vi "SVPO TDMS Write SGL Array (1 Ch).vi"(0 "tdms file":refnum<k34>, 1 "write channel properties? (T)":bool=TRUE, 5 "group name in":string="Waveform", 7 "channel name in":string="Channel0", 9 "scaled signal [EU]":sgl[](array[numeric]), 11 "sampling rate [Hz]":dbl=1.0, 12 "unit label":string) -> (4 "tdms file out":refnum<k34>, 6 "group name out":string, 8 "channel name out":string)   [LabVIEW 2017]
doc: "Writes single-precision waveform or scaled array data to the specified .tdms file in a format specific to the polymorphic instance. Use this VI on embedded targets that have limited computational resources. Wire data to the <B>scaled signal [EU]</B> input to determine the polymorphic instance to use or manually select the instance."
uses:
  <vilib>/addons/_NISVFA/_Shared subVIs/Controls/NI Channel Properties.ctl
  <vilib>/addons/_NISVFA/_Shared subVIs/Controls/LV Datatypes.ctl
  <vilib>/addons/_NISVFA/_Shared subVIs/Controls/svc_X-Axis Units.ctl
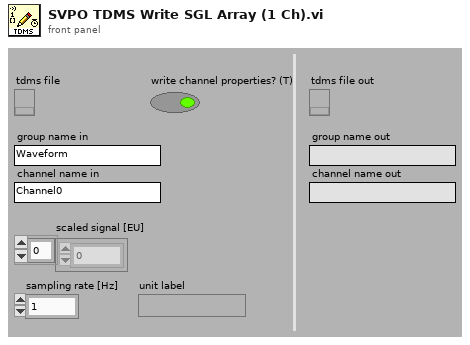
[diagram p1: front panel]
types:
  T1 = typedef "NI Channel Properties.ctl" = u16
  T2 = typedef "svc_X-Axis Units.ctl" = u16
  T3 = typedef "LV Datatypes.ctl" = i32
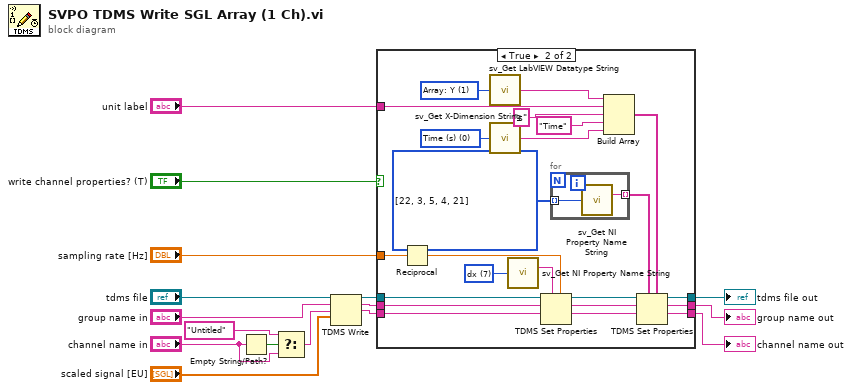
[diagram p0: block diagram]
diagram:
  n1 = Empty String/Path?(string/path="channel name in") -> (empty?=w16:bool)
  n2 = Select(t="Untitled" ("channel name"), s=w16, f="channel name in") -> (s? t:f=w8:string)
  n3 = TDMS Write(0:"tdms file", 5:"group name in", 7:w8, 9:"scaled signal [EU]") -> (4:w13:refnum<k34>, 6:w11:string, 8:w7:string)  [unwired: 2 in, 1 out]
  n4 = case shown="True" "write channel properties? (T)" {
    tunnel: [w19 w42] -> w5
    tunnel: w7 -> [w17 w39]
    tunnel: w11 -> [w18 w40]
    tunnel: w13 -> [w19 w41]
    tunnel: [w18 w33] -> w4
    tunnel: [w17 w34] -> w3
    tunnel: "sampling rate [Hz]" -> [_ w36]
    tunnel: "unit label" -> [_ w22]
    frame False {
    }
    frame True {
      w23 = T1[] [22, 3, 5, 4, 21] items=["Channel name", "Channel description", "Y-axis label", "Y-axis unit string", "X-axis label", "X-axis unit string", "x0", "dx", "Number of samples", "X channel", "Filter settled", "dB reference", "Window", "Window parameter", "Window size", "FFT size", "Peak units", "Spectrum type", "Magnitude scale", "Spectral density", "Sensor sensitivity (mV/EU)", "X-axis domain", "LabVIEW datatype"]
      w28 = T2 0 items=["Time (s)"=0, "Frequency-CB (Hz)"=1, "Frequency-CPB (Hz)"=1248, "Frequency-Arbitrary (Hz)"=2357, "Quefrency (s)"=2, "Revolutions (rev)"=3, "Order"=4, "Speed (RPM)"=11, "Speed (rad/s)"=21, "Index"=65535] ("x-axis units")
      w29 = T3 1 items=["String"=-2, "Boolean"=-1, "Scalar: y"=0, "Array: Y"=1, "Waveform: t0, dt, Y, variant"=2, "Cluster: x0, dx, Y"=3, "Cluster: X, Y"=4, "Waterfall"=5, "Colormap"=6] ("LabVIEW datatype")
      w37 = T1 7 items=["Channel name", "Channel description", "Axis label", "Unit string", "Waveform X-axis label", "Waveform X-axis unit string", "x0", "dx", "Number of samples", "X channel", "Filter settled", "dB reference", "Window", "Window parameter", "Window size", "FFT size", "Peak units", "Spectrum type", "Magnitude scale", "Spectral density", "Sensor sensitivity (mV/EU)", "X-axis dimension", "LabVIEW datatype", "Function type", "Function subtype", "X values", "Independent channel", "Column index", "Collection name", "Collection ID", "X Columns", "Phase unwrapped"] ("property")
      n5 = Reciprocal(x=w36) -> (1/x=w35:dbl)
      n6 = call <vilib>:"sv_Get LabVIEW Datatype String.vi"("LabVIEW datatype"=w29) -> ("datatype string"=w27:string)  [unwired: 4 in]
      n7 = call <vilib>:"sv_Get X-Dimension String.vi"("x-axis units"=w28) -> ("x-domain string"=w24:string)  [unwired: 4 in]
      n8 = call <vilib>:"sv_Get NI Property Name String.vi"("property"=w37) -> ("TDMS property name"=w38:string)  [unwired: 13 in, 1 out]
      n9 = TDMS Set Properties(5:w35, 7:w38, 9:w39, 10:w40, 11:w41) -> (1:w32:string, 2:w31:string, 3:w30:refnum<k34>)  [unwired: 1 in, 1 out]
      n10 = for {
        tunnel: [w44] -> w21 mode=indexing
        tunnel: w23 -> [w43] mode=indexing
        n11 = call <vilib>:"sv_Get NI Property Name String.vi"("property"=w43) -> ("TDMS property name"=w44:string)  [unwired: 13 in, 1 out]
      }
      n12 = Build Array(w27, w22, "s" ("group name"), "Time" ("channel name"), w24) -> (w20:string[])
      n13 = TDMS Set Properties(5:w20, 7:w21, 9:w32, 10:w31, 11:w30) -> (1:w34:string, 2:w33:string, 3:w42:refnum<k34>)  [unwired: 1 in, 1 out]
    }
  }
  "tdms file out" <- w5
  "channel name out" <- w3
  "group name out" <- w4
